vi "save_load_holos.vi"(8 "Phase rotation":dbl min=0.0 max=6.28318530718 step=0.01570796326, 11 "output cluster":T5 {"SLM Settings - A"."Resolution x" format="%#.0f"; "SLM Settings - A"."SLM width (m)" format="%_6f"; "SLM Settings - A"."SLM height (m)" format="%#_6f"}) -> (0 "holo grayscale":dbl[][](array[numeric]), 3 "appended path":path, 4 "Loaded?":bool)   [LabVIEW 2020]
uses:
  typeDefs/BPandSLM.ctl
  typeDefs/beamData.ctl
  typeDefs/modesArray.ctl
  typeDefs/modeCluster.ctl
  <vilib>/Utility/file.llb/Read Delimited Spreadsheet (DBL).vi
panel:
  out "error out":errorcluster
  out "resulting string":string
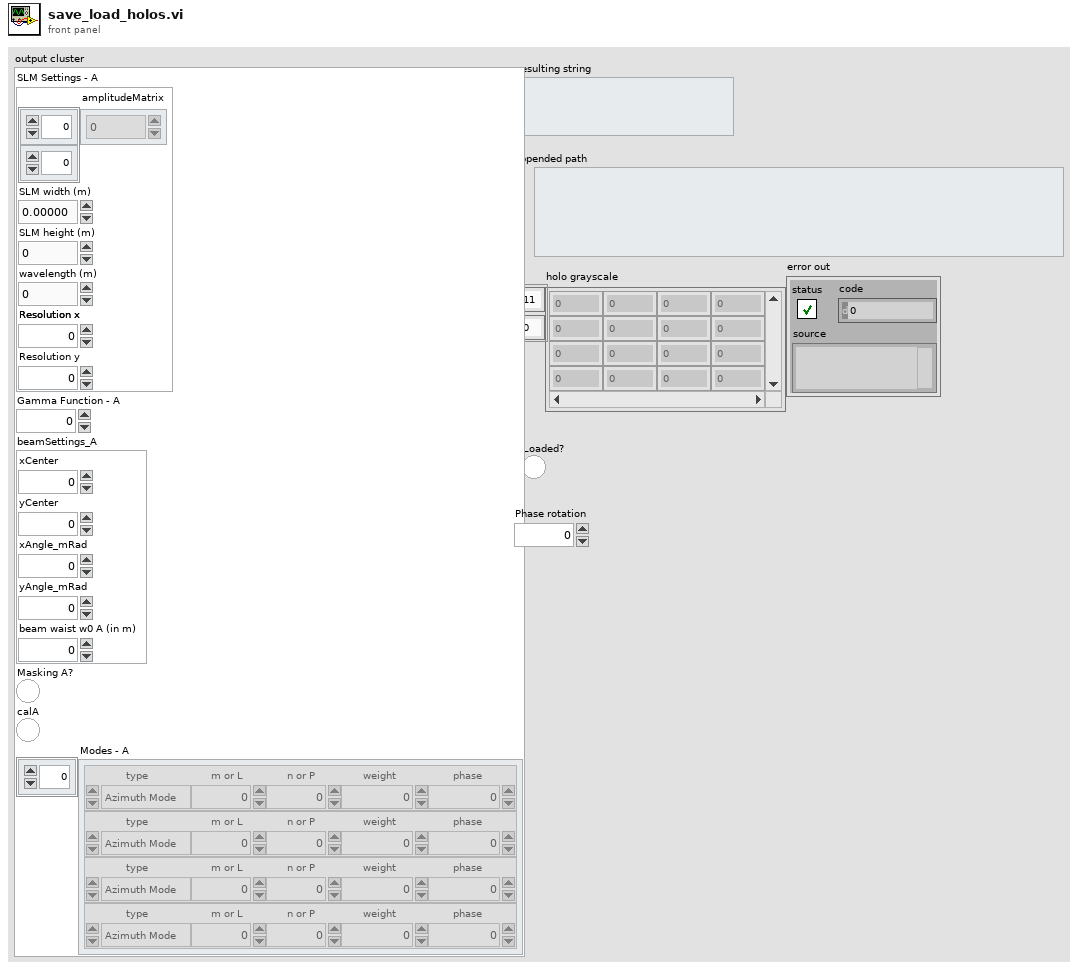
[diagram p1: front panel]
types:
  T1 = typedef "BPandSLM.ctl" = cluster{"amplitudeMatrix":csg[][], "SLM width (m)":dbl, "SLM height (m)":dbl, "wavelength (m)":dbl, "Resolution x":u32, "Resolution y":u32}
  T2 = typedef "beamData.ctl" = cluster{"xCenter":dbl, "yCenter":dbl, "xAngle_mRad":dbl, "yAngle_mRad":dbl, "beamWaist":dbl}
  T3 = typedef "modesArray.ctl" = T4[]
  T4 = typedef "modeCluster.ctl" = cluster{"type":enum16{"Azimuth Mode", "LG Mode", "HG Mode", "Pixel"}, "m or L":i32, "n or P":i32, "weight":dbl, "phase":dbl}
  T5 = cluster{"SLM Settings - A":T1, "Gamma Function - A":dbl, "beamSettings_A":T2, "Masking A?":bool, "calA":bool, "Modes - A":T3}
  T6 = enum16{"Azimuth Mode", "LG Mode", "HG Mode", "Pixel"}
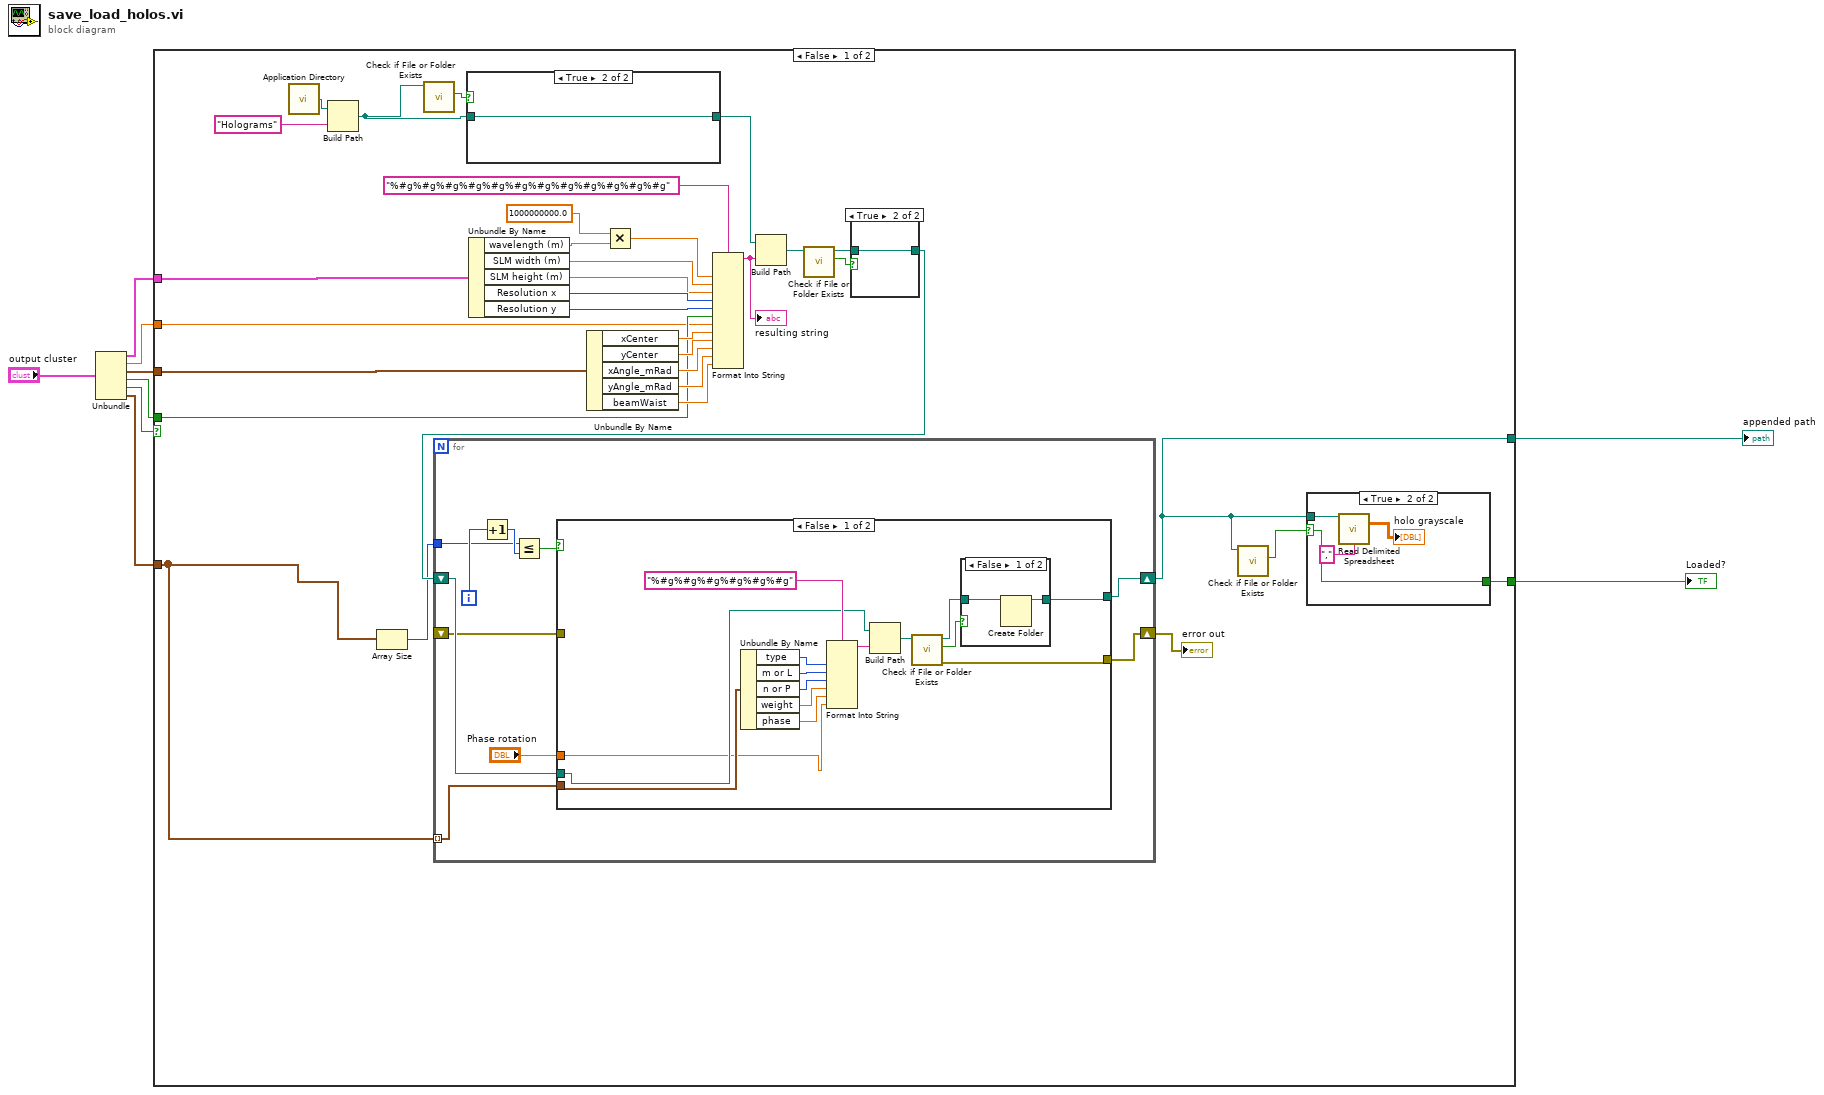
[diagram p0: block diagram]
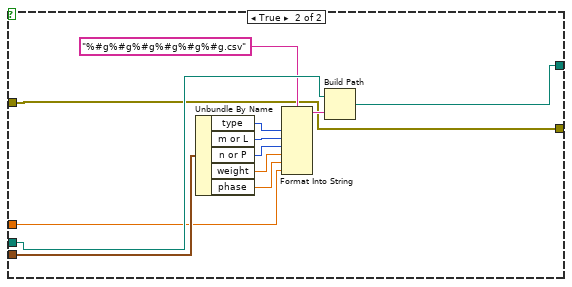
[diagram p4: hidden frame]
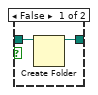
[diagram p5: hidden frame]
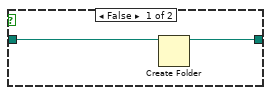
[diagram p6: hidden frame]
diagram:
  n1 = Unbundle("output cluster") -> ("SLM Settings - A"=w6:T1, "Gamma Function - A"=w3:dbl, "beamSettings_A"=w2:T2, "Masking A?"=w4:bool, "calA"=w5:bool, "Modes - A"=w1:T3)
  n2 = case shown="False" w5 {
    tunnel: [w11 _] -> w9
    tunnel: [w22 _] -> w8
    tunnel: w6 -> [w21 _]
    tunnel: w4 -> [w20 _]
    tunnel: w3 -> [w19 _]
    tunnel: w2 -> [w18 _]
    tunnel: w1 -> [w13 _]
    frame False {
      n3 = call <vilib>:"Application Directory.vi"() -> ("Application Directory"=w42:path)
      n4 = Build Path(base path=w42, name or relative path="Holograms") -> (appended path=w39:path)
      n5 = Array Size(array=w13) -> (size(s)=w12:i32)
      n6 = call <vilib>:"Check if File or Folder Exists.vi"("path"=w39) -> ("file or folder exists?"=w40:bool)  [unwired: 8 in, 2 out]
      n7 = case shown="True" w40 {
        tunnel: w39 -> [w91 w92]
        tunnel: [w90 w92] -> w34
        frame False {
          n8 = Create Folder(path (use dialog)=w91) -> (created path=w90:path)  [unwired: 2 in, 2 out]
        }
        frame True {
        }
      }
      n9 = Unbundle By Name(w21) -> ("wavelength (m)"=w30:dbl, "SLM width (m)"=w38:dbl, "SLM height (m)"=w28:dbl, "Resolution x"=w37:u32, "Resolution y"=w36:u32)
      n10 = Unbundle By Name(w18) -> ("xCenter"=w27:dbl, "yCenter"=w26:dbl, "xAngle_mRad"=w25:dbl, "yAngle_mRad"=w24:dbl, "beamWaist"=w23:dbl)
      n11 = Multiply(x=1000000000.0 ("y"), y=w30) -> (x*y=w35:dbl)
      n12 = Format Into String(format string="%#g%#g%#g%#g%#g%#g%#g%#g%#g%#g%#g%#g", w35, w38, w28, w37, w36, w20, w19, w27, w26, w25, w24, w23) -> (resulting string=w33:string)  [unwired: 2 in, 1 out]
      "resulting string" <- w33
      n13 = Build Path(base path=w34, name or relative path=w33) -> (appended path=w31:path)
      n14 = call <vilib>:"Check if File or Folder Exists.vi"("path"=w31) -> ("file or folder exists?"=w32:bool, "dup path"=w16:path)  [unwired: 8 in, 1 out]
      n15 = case shown="True" w32 {
        tunnel: w16 -> [w88 w89]
        tunnel: [w87 w89] -> w15
        frame False {
          n16 = Create Folder(path (use dialog)=w88) -> (created path=w87:path)  [unwired: 2 in, 2 out]
        }
        frame True {
        }
      }
      n17 = for {
        tunnel: w13 -> [w51] mode=indexing
        shift-right: [w50] -> w11
        shift-left: w15 -> [w52]
        tunnel: w12 -> [w54]
        shift-right: [w49] -> w14
        shift-left: _ -> [w48]
        i -> [w56]
        n18 = Increment(x=w56) -> (x+1=w55:i32)
        n19 = Less Or Equal?(x=w54, y=w55) -> (x <= y?=w53:bool)
        n20 = case shown="False" w53 {
          tunnel: w52 -> [w62 w80]
          tunnel: w51 -> [w61 w78]
          tunnel: [w60 w76] -> w50
          tunnel: [w58 w77] -> w49
          tunnel: w48 -> [_ w77]
          tunnel: "Phase rotation" -> [w57 w75]
          frame False {
            n21 = Unbundle By Name(w61) -> ("type"=w64:T6, "m or L"=w67:i32, "n or P"=w65:i32, "weight"=w66:dbl, "phase"=w68:dbl)
            n22 = Format Into String(format string="%#g%#g%#g%#g%#g%#g", w64, w67, w65, w66, w68, w57) -> (resulting string=w70:string)  [unwired: 2 in, 1 out]
            n23 = Build Path(base path=w62, name or relative path=w70) -> (appended path=w69:path)
            n24 = call <vilib>:"Check if File or Folder Exists.vi"("path"=w69) -> ("error out"=w58:errorcluster, "file or folder exists?"=w59:bool, "dup path"=w71:path)  [unwired: 8 in]
            n25 = case shown="False" w59 {
              tunnel: [w73 w74] -> w60
              tunnel: w71 -> [w72 w74]
              frame False {
                n26 = Create Folder(path (use dialog)=w72) -> (created path=w73:path)  [unwired: 2 in, 2 out]
              }
              frame True {
              }
            }
          }
          frame True {
            n27 = Unbundle By Name(w78) -> ("type"=w81:T6, "m or L"=w84:i32, "n or P"=w82:i32, "weight"=w83:dbl, "phase"=w85:dbl)
            n28 = Format Into String(format string="%#g%#g%#g%#g%#g%#g.csv", w81, w84, w82, w83, w85, w75) -> (resulting string=w86:string)  [unwired: 2 in, 1 out]
            n29 = Build Path(base path=w80, name or relative path=w86) -> (appended path=w76:path)
          }
        }
      }
      "error out" <- w14
      n30 = call <vilib>:"Check if File or Folder Exists.vi"("path"=w11) -> ("file or folder exists?"=w10:bool)  [unwired: 8 in, 2 out]
      n31 = case shown="True" w10 {
        selector: w10 -> [_ w44]
        tunnel: w11 -> [_ w46]
        tunnel: [_ w44] -> w22
        frame False {
        }
        frame True {
          n32 = call-poly <vilib>:"Read Delimited Spreadsheet.vi"("file path (dialog if empty)"=w46, "delimiter (\\t)"="," ("delimiter (\\t)")) -> ("all rows"=→"holo grayscale":dbl[][])  [unwired: 8 in, 5 out]
        }
      }
    }
    frame True {
    }
  }
  "appended path" <- w9
  "Loaded?" <- w8
